vi "XW_Linearise_+_temp_comp.vi"(5 "Calib const":dbl[](array[numeric]) format="%.4f", 6 "XW2 voltage":dbl[](array[numeric]) format="%.4f", 7 "XW1 voltage":dbl[](array[numeric]) format="%.4f") -> (0 "U1":dbl[](array[numeric]) format="%.2f", 1 "V":dbl[](array[numeric]) format="%.2f", 2 "U2":dbl[](array[numeric]) format="%.2f", 3 "U":dbl[](array[numeric]) format="%.2f")   [LabVIEW 2011]
uses:
  XW calib map/XW_Map_Global.vi
  Globals/Meas_global.vi
  Globals/Dynamic_call_global.ph.vi
  <vilib>/Analysis/NI_AALBase.lvlib
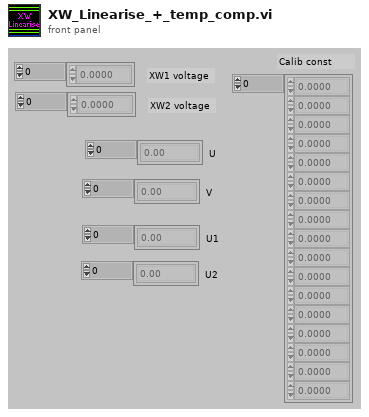
[diagram p1: front panel]
types:
  T1 = cluster{"Calib const[0]":dbl, "Calib const[1]":dbl, "Calib const[2]":dbl, "Calib const[3]":dbl, "Calib const[4]":dbl, "Calib const[5]":dbl, "Calib const[6]":dbl, "Calib const[7]":dbl, "Calib const[8]":dbl, "Calib const[9]":dbl, "Calib const[10]":dbl, "Calib const[11]":dbl, "Calib const[12]":dbl, "Calib const[13]":dbl, "Calib const[14]":dbl, "Calib const[15]":dbl, "Calib const[16]":dbl, "Calib const[17]":dbl}
  T2 = typedef "Map method.ctl" = enum16{"Triangle mesh", "Polynomial surface", "Const. Psi_eff (std.)", "Psi_eff = f(Umagn.)", "Psi_eff, k = f(Umagn.)"}
  T3 = typedef "Trimmed down TreeNode2D.ctl" = cluster{"Xmax":dbl, "Xmin":dbl, "Ymax":dbl, "Ymin":dbl, "Xc":dbl, "Yc":dbl, "ObjIndexList":i32[], "NodeQ1Index":i32, "NodeQ2Index":i32, "NodeQ3Index":i32, "NodeQ4Index":i32}
  T4 = typedef "Triangle2D.ctl" = cluster{"V10":dbl[], "V20":dbl[], "1/det":dbl, "V0":cluster{"PosVector":dbl[], "ValueVector":dbl[]}, "V1":cluster{"PosVector":dbl[], "ValueVector":dbl[]}, "V2":cluster{"PosVector":dbl[], "ValueVector":dbl[]}, "V21":dbl[]}
  T5 = enum16{"2nd component as calculated", "2nd component multipled by -1"}
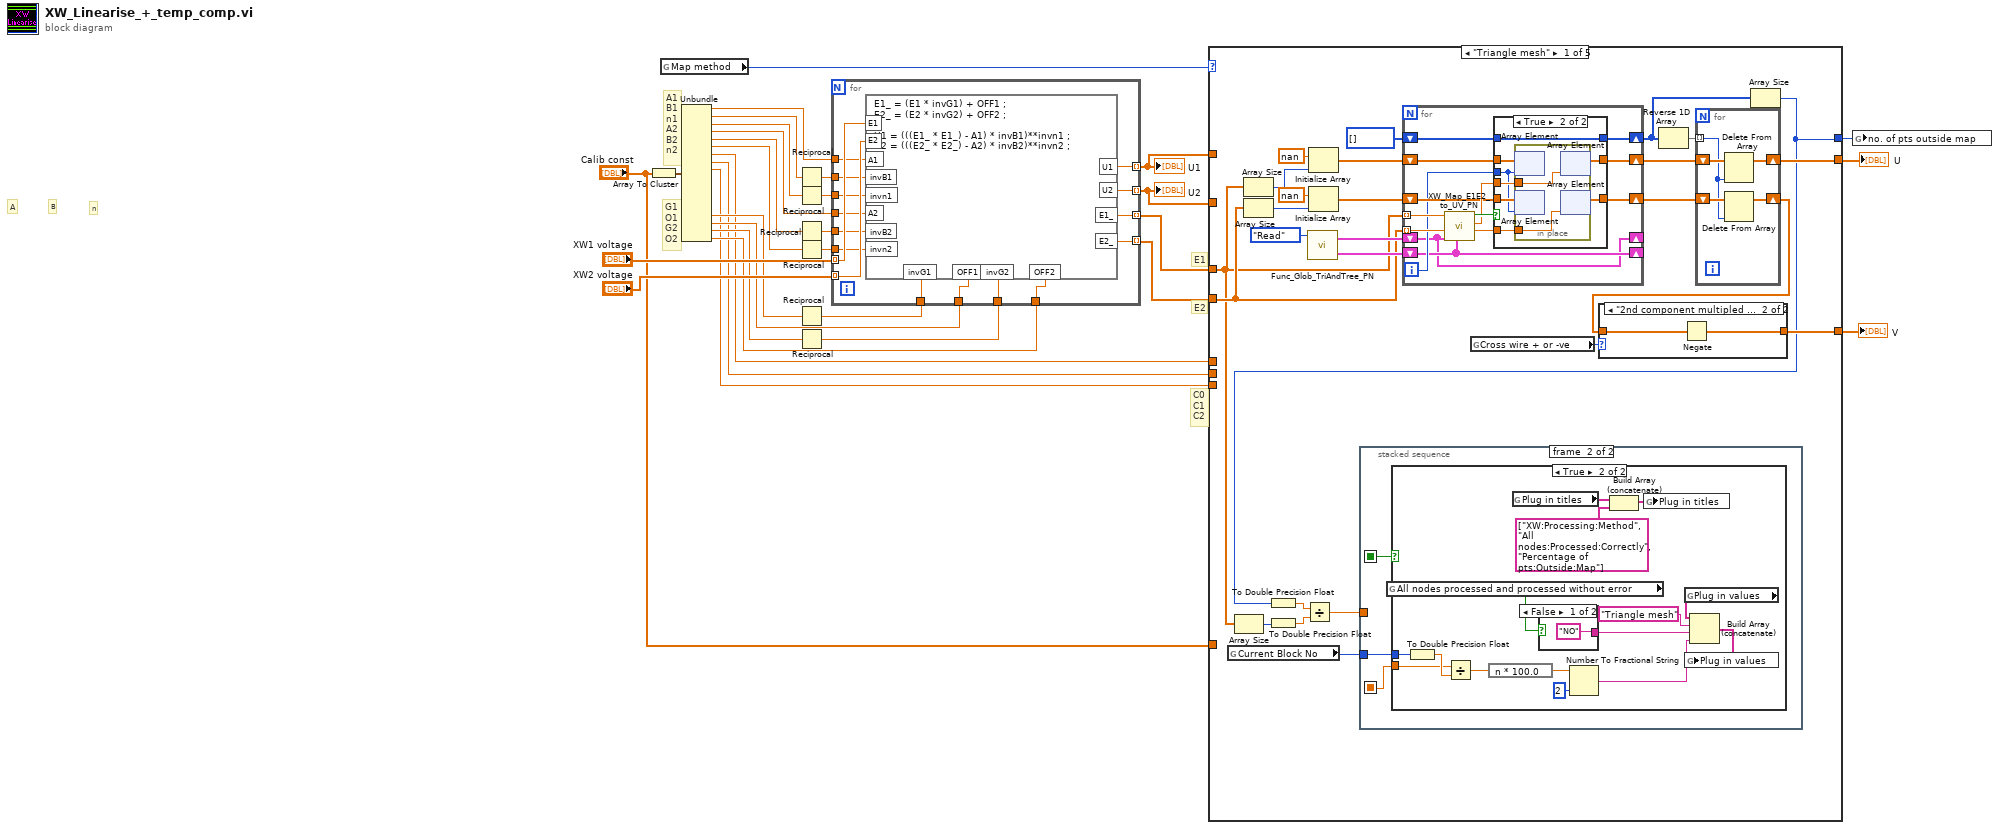
[diagram p0: block diagram]
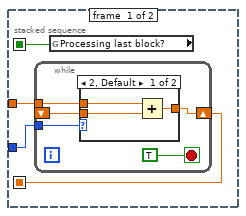
[diagram p2: hidden frame]
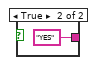
[diagram p5: hidden frame]
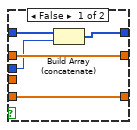
[diagram p6: hidden frame]
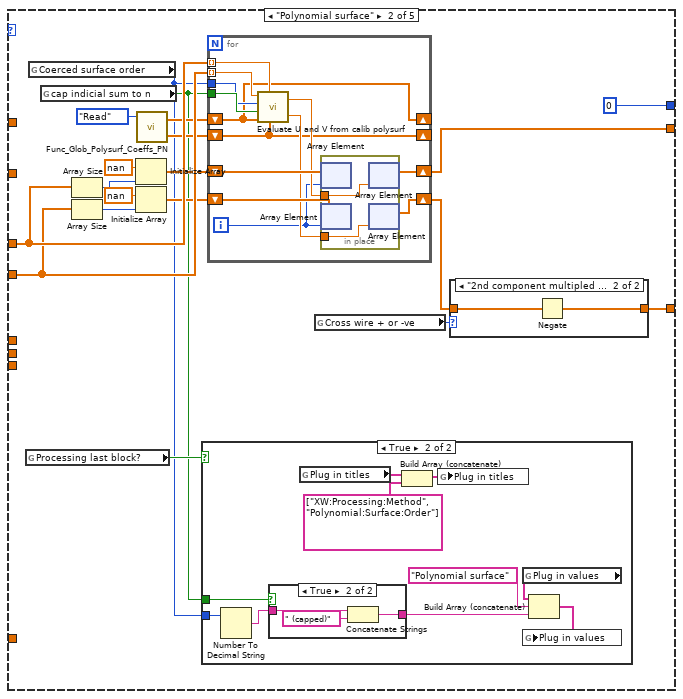
[diagram p8: hidden frame]
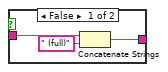
[diagram p10: hidden frame]
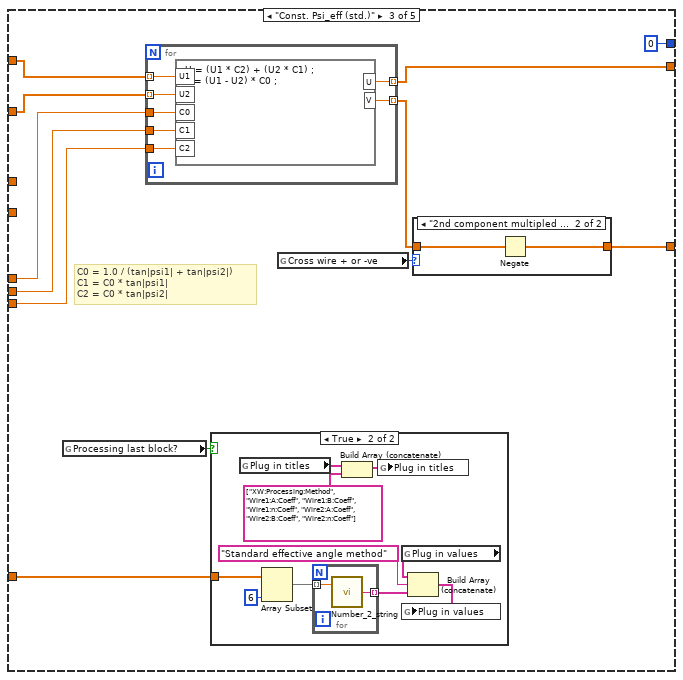
[diagram p12: hidden frame]
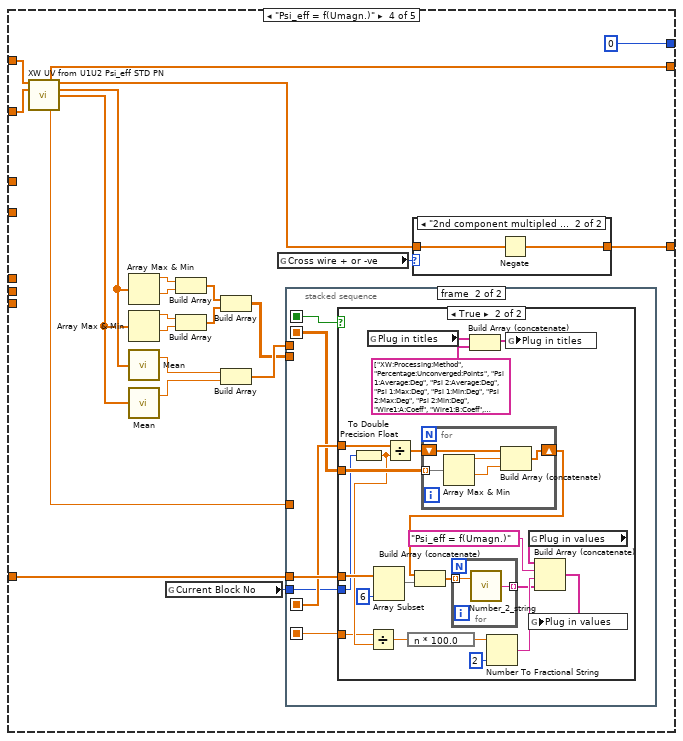
[diagram p15: hidden frame]
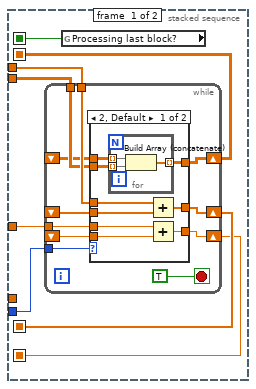
[diagram p16: hidden frame]
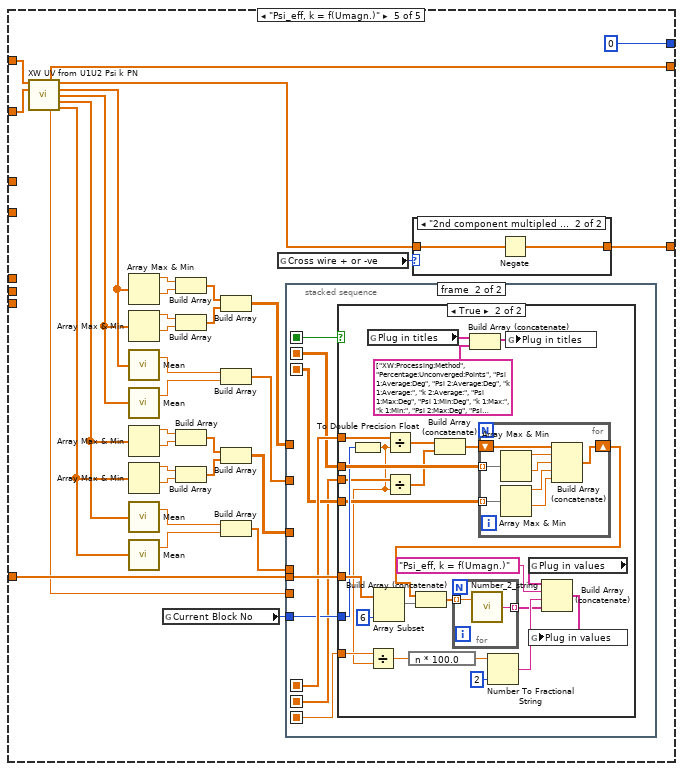
[diagram p20: hidden frame]
diagram:
  # "C0\nC1\nC2"
  # "E2"
  # "E1"
  # "G1\nO1\nG2\nO2"
  # "A1\nB1\nn1\nA2\nB2\nn2"
  # "n"
  # "B"
  # "A"
  n1 = Array To Cluster(array="Calib const") -> (cluster=w31:T1)
  n2 = global read "XW_Map_Global.vi" "Map method"() -> (w28:T2)
  n3 = Unbundle(w31) -> ("Calib const[0]"=w22:dbl, "Calib const[1]"=w16:dbl, "Calib const[2]"=w12:dbl, "Calib const[3]"=w21:dbl, "Calib const[4]"=w14:dbl, "Calib const[5]"=w10:dbl, "Calib const[6]"=w3:dbl, "Calib const[7]"=w2:dbl, "Calib const[8]"=w1:dbl, "Calib const[14]"=w8:dbl, "Calib const[15]"=w19:dbl, "Calib const[16]"=w6:dbl, "Calib const[17]"=w20:dbl)  [unwired: 5 out]
  n4 = Reciprocal(x=w16) -> (1/x=w15:dbl)
  n5 = Reciprocal(x=w12) -> (1/x=w11:dbl)
  n6 = Reciprocal(x=w14) -> (1/x=w13:dbl)
  n7 = Reciprocal(x=w10) -> (1/x=w9:dbl)
  n8 = Reciprocal(x=w8) -> (1/x=w7:dbl)
  n9 = Reciprocal(x=w6) -> (1/x=w5:dbl)
  n10 = for {
    tunnel: [w47] -> w26 mode=indexing
    tunnel: [w46] -> w25 mode=indexing
    tunnel: [w45] -> w18 mode=indexing
    tunnel: [w44] -> w17 mode=indexing
    tunnel: "XW1 voltage" -> [w43] mode=indexing
    tunnel: "XW2 voltage" -> [w42] mode=indexing
    tunnel: w22 -> [w41]
    tunnel: w15 -> [w40]
    tunnel: w11 -> [w39]
    tunnel: w21 -> [w38]
    tunnel: w13 -> [w37]
    tunnel: w9 -> [w36]
    tunnel: w20 -> [w35]
    tunnel: w5 -> [w34]
    tunnel: w19 -> [w33]
    tunnel: w7 -> [w32]
    n11 = formula code="E1_ = (E1 * invG1) + OFF1 ;\nE2_ = (E2 * invG2) + OFF2 ;\n\nU1 = (((E1_ * E1_) - A1) * invB1)**invn1 ;\nU2 = (((E2_ * E2_) - A2) * invB2)**invn2 ;"("E1"=w43, "E2"=w42, "A1"=w41, "invB1"=w40, "invn1"=w39, "A2"=w38, "invB2"=w37, "invn2"=w36, "invG1"=w32, "OFF1"=w33, "invG2"=w34, "OFF2"=w35) -> ("E1_"=w47:dbl, "E2_"=w46:dbl, "U1"=w45:dbl, "U2"=w44:dbl)
  }
  "U2" <- w17
  "U1" <- w18
  n12 = case shown="\"Triangle mesh\"" w28 {
    tunnel: w25 -> [w54 w155 _ _ _]
    tunnel: w26 -> [w50 w156 _ _ _]
    tunnel: [w60 w152 w204 w250 w355] -> w30
    tunnel: [w73 w162 w206 w236 w352] -> w29
    tunnel: [w55 0 0 0 0] -> w27
    tunnel: w18 -> [_ _ w203 w252 w357]
    tunnel: w17 -> [_ _ w202 w251 w356]
    tunnel: "Calib const" -> [_ _ w198 w232 w338]
    tunnel: w3 -> [_ _ w201 _ _]
    tunnel: w2 -> [_ _ w200 _ _]
    tunnel: w1 -> [_ _ w199 _ _]
    frame "Triangle mesh" {
      n13 = global read "Meas_global.vi" "Current Block No"() -> (w49:i32)
      n14 = Array Size(array=w50) -> (size(s)=w53:i32)
      n15 = Array Size(array=w50) -> (size(s)=w69:i32)
      n16 = Array Size(array=w54) -> (size(s)=w68:i32)
      n17 = To Double Precision Float(number=w53) -> (double precision float=w51:dbl)
      n18 = call "Func_Glob_TriAndTree_PN.vi"("Action"=enum16{"Read", "Write"}."Read") -> ("Trimmed down TreeNode array OUT"=w56:T3[], "Corrected triangles OUT"=w57:T4[])  [unwired: 2 in]
      n19 = Initialize Array(nan ("element"), w69) -> (w66:dbl[])
      n20 = Initialize Array(nan ("element"), w68) -> (w67:dbl[])
      n21 = for {
        tunnel: w50 -> [w125] mode=indexing
        tunnel: w54 -> [w124] mode=indexing
        shift-right: [w113] -> w59
        shift-left: i32[] [] -> [w112]
        shift-right: [w120] -> w64
        shift-left: w66 -> [w119]
        shift-right: [w117] -> w63
        shift-left: w67 -> [w118]
        shift-right: [w114] -> _
        shift-left: w57 -> [w114]
        shift-right: [w115] -> _
        shift-left: w56 -> [w115]
        i -> [w116]
        n22 = call "XW_Map_E1E2_to_UV_PN.vi"("Trimmed down TreeNode array"=w115, "Triangulated XW Calib Map Mesh"=w114, "(E2 / G2) + O2 (Volts)"=w124, "(E1 / G1) + O1 (Volts)"=w125) -> ("V (m/s)"=w121:dbl, "U (m/s)"=w122:dbl, "Voltages are inside calibrated region"=w123:bool)  [unwired: 5 out]
        n23 = case shown="True" w123 {
          tunnel: w122 -> [_ w134]
          tunnel: w112 -> [w126 w138]
          tunnel: [w127 w138] -> w113
          tunnel: w121 -> [_ w133]
          tunnel: [w130 w136] -> w120
          tunnel: w119 -> [w130 w137]
          tunnel: w118 -> [w129 w135]
          tunnel: [w129 w132] -> w117
          tunnel: w116 -> [w128 w131]
          frame False {
            n24 = Build Array (concatenate)(w126, w128) -> (w127:i32[])
          }
          frame True {
            n25 = in-place {
              in-place-border: w134 -> [w140]
              in-place-border: w133 -> [w139]
              n26 = in-place-array #1(w137, w131) -> ()  [unwired: 1 out]
              n27 = in-place-array #2(w135, w131) -> ()  [unwired: 1 out]
              n28 = in-place-array #1(w140) -> (w136:dbl[])  [unwired: 1 out]
              n29 = in-place-array #2(w139) -> (w132:dbl[])  [unwired: 1 out]
            }
          }
        }
      }
      n30 = global read "Meas_global.vi" "Cross wire + or -ve"() -> (w72:T5)
      n31 = Reverse 1D Array(array=w59) -> (reversed array=w62:i32[])
      n32 = for {
        shift-right: [w108] -> w60
        shift-left: w64 -> [w111]
        shift-right: [w109] -> w61
        shift-left: w63 -> [w110]
        tunnel: w62 -> [w107] mode=indexing
        n33 = Delete From Array(array=w111, index=w107) -> (array with subset deleted=w108:dbl[])  [unwired: 1 in, 1 out]
        n34 = Delete From Array(array=w110, index=w107) -> (array with subset deleted=w109:dbl[])  [unwired: 1 in, 1 out]
      }
      n35 = case shown="\"2nd component multipled by -1\"" w72 {
        tunnel: [w141 w143] -> w73
        tunnel: w61 -> [w141 w142]
        frame "2nd component as calculated" {
        }
        frame "2nd component multipled by -1" {
          n36 = Negate(x=w142) -> (-x=w143:dbl[])
        }
      }
      n37 = Array Size(array=w59) -> (size(s)=w55:i32)
      n38 = To Double Precision Float(number=w55) -> (double precision float=w52:dbl)
      n39 = Divide(x=w52, y=w51) -> (x/y=w48:dbl)
      n40 = stacked-sequence {
        seq-local: [w77 _] -> [_ w87]
        seq-local: [w76 _] -> [_ w89]
        tunnel: w49 -> [w75 w88]
        tunnel: w48 -> [w74 _]
        frame #0 {
          n41 = while {
            shift-right: [w82] -> w77
            shift-left: _ -> [w79]
            tunnel: w75 -> [w80]
            tunnel: w74 -> [w78]
            stop <- TRUE stop-if-true
            n42 = case shown="2, Default" w80 {
              tunnel: w79 -> [w84 _]
              tunnel: [w85 w86] -> w82
              tunnel: w78 -> [w83 w86]
              frame 2, Default {
                n43 = Add(x=w83, y=w84) -> (x+y=w85:dbl)
              }
              frame 1 {
              }
            }
          }
          n44 = global read "Meas_global.vi" "Processing last block?"() -> (w76:bool)
        }
        frame #1 {
          n45 = case shown="True" w89 {
            tunnel: w88 -> [_ w104]
            tunnel: w87 -> [_ w101]
            frame False {
            }
            frame True {
              n46 = global read "XW_Map_Global.vi" "All nodes processed and processed without error"() -> (w99:bool)
              n47 = To Double Precision Float(number=w104) -> (double precision float=w102:dbl)
              n48 = Divide(x=w101, y=w102) -> (x/y=w91:dbl)
              n49 = expression code="n * 100.0"(w91) -> (w90:dbl)
              n50 = global read "Dynamic_call_global.ph.vi" "Plug in titles"() -> (w95:string[])
              n51 = case shown="False" w99 {
                tunnel: ["NO" "YES"] -> w100
                frame False {
                }
                frame True {
                }
              }
              n52 = Number To Fractional String(number=w90, precision (6)=i16 2) -> (F-format string=w92:string)  [unwired: 2 out]
              n53 = Build Array (concatenate)(w95, string[] ["XW:Processing:Method", "All nodes:Processed:Correctly", "Percentage of pts:Outside:Map"] ("array")) -> (w93:string[])
              n54 = global write "Dynamic_call_global.ph.vi" "Plug in titles"(w93) -> ()
              n55 = global read "Dynamic_call_global.ph.vi" "Plug in values"() -> (w97:string[])
              n56 = Build Array (concatenate)(w97, "Triangle mesh", w100, w92) -> (w94:string[])
              n57 = global write "Dynamic_call_global.ph.vi" "Plug in values"(w94) -> ()
            }
          }
        }
      }
    }
    frame "Polynomial surface" {
      n58 = global read "Meas_global.vi" "Processing last block?"() -> (w146:bool)
      n59 = global read "XW_Map_Global.vi" "Coerced surface order"() -> (w145:i32)
      n60 = global read "XW_Map_Global.vi" "cap indicial sum to n"() -> (w144:bool)
      n61 = Array Size(array=w156) -> (size(s)=w158:i32)
      n62 = Array Size(array=w155) -> (size(s)=w157:i32)
      n63 = Initialize Array(nan ("element"), w158) -> (w154:dbl[])
      n64 = Initialize Array(nan ("element"), w157) -> (w153:dbl[])
      n65 = call "Func_Glob_Polysurf_Coeffs_PN.vi"("Action"=enum16{"Read", "Write"}."Read") -> ("alpha(rad) coeffs OUT"=w148:dbl[], "Ucal coeffs OUT"=w149:dbl[])  [unwired: 2 in]
      n66 = case shown="True" w146 {
        tunnel: w145 -> [_ w165]
        tunnel: w144 -> [_ w163]
        frame False {
        }
        frame True {
          n67 = Number To Decimal String(number=w165) -> (decimal integer string=w164:string)  [unwired: 1 out]
          n68 = case shown="True" w163 {
            tunnel: [w173 w176] -> w166
            tunnel: w164 -> [w175 w178]
            frame False {
              n69 = Concatenate Strings(w175, " (full)") -> (w173:string)
            }
            frame True {
              n70 = Concatenate Strings(w178, " (capped)") -> (w176:string)
            }
          }
          n71 = global read "Dynamic_call_global.ph.vi" "Plug in titles"() -> (w170:string[])
          n72 = Build Array (concatenate)(w170, string[] ["XW:Processing:Method", "Polynomial:Surface:Order"] ("array")) -> (w172:string[])
          n73 = global write "Dynamic_call_global.ph.vi" "Plug in titles"(w172) -> ()
          n74 = global read "Dynamic_call_global.ph.vi" "Plug in values"() -> (w168:string[])
          n75 = Build Array (concatenate)(w168, "Polynomial surface", w166) -> (w171:string[])
          n76 = global write "Dynamic_call_global.ph.vi" "Plug in values"(w171) -> ()
        }
      }
      n77 = for {
        tunnel: w156 -> [w191] mode=indexing
        tunnel: w155 -> [w190] mode=indexing
        tunnel: w144 -> [w189]
        shift-right: [w187] -> w151
        shift-left: w153 -> [w185]
        shift-right: [w188] -> w152
        shift-left: w154 -> [w186]
        tunnel: w145 -> [w181]
        shift-right: [w180] -> _
        shift-left: w148 -> [w180]
        shift-right: [w179] -> _
        shift-left: w149 -> [w179]
        i -> [w182]
        n78 = call "Evaluate U and V from calib polysurf.vi"("alpha(rad) coeffs"=w180, "E1 / G1 + O1"=w191, "Ucal coeffs"=w179, "cap indicial sum to n"=w189, "surface order (n)"=w181, "E2 / G2 + O2"=w190) -> ("V (m/s)"=w184:dbl, "U (m/s)"=w183:dbl)
        n79 = in-place {
          in-place-border: w183 -> [w193]
          in-place-border: w184 -> [w192]
          n80 = in-place-array #3(w186, w182) -> ()  [unwired: 1 out]
          n81 = in-place-array #4(w185, w182) -> ()  [unwired: 1 out]
          n82 = in-place-array #3(w193) -> (w188:dbl[])  [unwired: 1 out]
          n83 = in-place-array #4(w192) -> (w187:dbl[])  [unwired: 1 out]
        }
      }
      n84 = global read "Meas_global.vi" "Cross wire + or -ve"() -> (w161:T5)
      n85 = case shown="\"2nd component multipled by -1\"" w161 {
        tunnel: [w194 w196] -> w162
        tunnel: w151 -> [w194 w195]
        frame "2nd component as calculated" {
        }
        frame "2nd component multipled by -1" {
          n86 = Negate(x=w195) -> (-x=w196:dbl[])
        }
      }
    }
    frame "Const. Psi_eff (std.)" {
      # "C0 = 1.0 / (tan|psi1| + tan|psi2|)\nC1 = C0 * tan|psi1|\nC2 = C0 * tan|psi2|"
      n87 = global read "Meas_global.vi" "Processing last block?"() -> (w197:bool)
      n88 = for {
        tunnel: [w227] -> w205 mode=indexing
        tunnel: [w226] -> w204 mode=indexing
        tunnel: w203 -> [w225] mode=indexing
        tunnel: w202 -> [w224] mode=indexing
        tunnel: w201 -> [w223]
        tunnel: w200 -> [w222]
        tunnel: w199 -> [w221]
        n89 = formula code="U = (U1 * C2) + (U2 * C1) ;\nV = (U1 - U2) * C0 ;"("U1"=w225, "U2"=w224, "C1"=w222, "C2"=w221, "C0"=w223) -> ("U"=w226:dbl, "V"=w227:dbl)
      }
      n90 = case shown="True" w197 {
        tunnel: w198 -> [_ w212]
        frame False {
        }
        frame True {
          n91 = global read "Dynamic_call_global.ph.vi" "Plug in titles"() -> (w216:string[])
          n92 = Array Subset(array=w212, length=6) -> (w211:dbl[])  [unwired: 1 in]
          n93 = for {
            tunnel: w211 -> [w220] mode=indexing
            tunnel: [w219] -> w215 mode=indexing
            n94 = call "Number_2_string.vi"("number"=w220) -> ("String"=w219:string)  [unwired: 1 in]
          }
          n95 = Build Array (concatenate)(w216, string[] ["XW:Processing:Method", "Wire1:A:Coeff", "Wire1:B:Coeff", "Wire1:n:Coeff", "Wire2:A:Coeff", "Wire2:B:Coeff", "Wire2:n:Coeff"] ("array")) -> (w218:string[])
          n96 = global write "Dynamic_call_global.ph.vi" "Plug in titles"(w218) -> ()
          n97 = global read "Dynamic_call_global.ph.vi" "Plug in values"() -> (w210:string[])
          n98 = Build Array (concatenate)(w210, "Standard effective angle method", w215) -> (w217:string[])
          n99 = global write "Dynamic_call_global.ph.vi" "Plug in values"(w217) -> ()
        }
      }
      n100 = global read "Meas_global.vi" "Cross wire + or -ve"() -> (w207:T5)
      n101 = case shown="\"2nd component multipled by -1\"" w207 {
        tunnel: [w228 w230] -> w206
        tunnel: w205 -> [w228 w229]
        frame "2nd component as calculated" {
        }
        frame "2nd component multipled by -1" {
          n102 = Negate(x=w229) -> (-x=w230:dbl[])
        }
      }
    }
    frame "Psi_eff = f(Umagn.)" {
      n103 = call "XW UV from U1U2 Psi_eff STD PN.vi"("U1cal (m/s)"=w252, "U2cal (m/s)"=w251) -> ("U (m/s)"=w250:dbl[], "V (m/s)"=w237:dbl[], "Psi1 (deg)"=w248:dbl[], "Psi2 (deg)"=w247:dbl[], "Unconverged points (fraction)"=w231:dbl)  [unwired: 9 out]
      n104 = Array Max & Min(array=w248) -> (max value=w243:dbl, min value=w244:dbl)  [unwired: 2 out]
      n105 = Array Max & Min(array=w247) -> (max value=w242:dbl, min value=w241:dbl)  [unwired: 2 out]
      n106 = call <vilib>:"Mean.vi"("X"=w248) -> ("mean"=w246:dbl)  [unwired: 1 out]
      n107 = call <vilib>:"Mean.vi"("X"=w247) -> ("mean"=w245:dbl)  [unwired: 1 out]
      n108 = global read "Meas_global.vi" "Current Block No"() -> (w235:i32)
      n109 = Build Array(w243, w244) -> (w239:dbl[])
      n110 = Build Array(w242, w241) -> (w240:dbl[])
      n111 = Build Array(w239, w240) -> (w233:dbl[][])
      n112 = Build Array(w246, w245) -> (w234:dbl[])
      n113 = global read "Meas_global.vi" "Cross wire + or -ve"() -> (w238:T5)
      n114 = stacked-sequence {
        seq-local: [w258 _] -> [_ w291]
        seq-local: [w256 _] -> [_ w289]
        seq-local: [w257 _] -> [_ w290]
        seq-local: [w253 _] -> [_ w287]
        tunnel: w234 -> [w260 _]
        tunnel: w233 -> [w259 _]
        tunnel: w232 -> [_ w292]
        tunnel: w235 -> [w255 w288]
        tunnel: w231 -> [w254 _]
        frame #0 {
          n115 = while {
            shift-right: [w269] -> w258
            shift-left: _ -> [w270]
            tunnel: w260 -> [w271]
            shift-right: [w267] -> w256
            shift-left: _ -> [w265]
            tunnel: w259 -> [w266]
            tunnel: w255 -> [w264]
            shift-right: [w261] -> w253
            shift-left: _ -> [w263]
            tunnel: w254 -> [w262]
            stop <- TRUE stop-if-true
            n116 = case shown="2, Default" w264 {
              tunnel: w271 -> [w280 w286]
              tunnel: w270 -> [w279 _]
              tunnel: [w278 w286] -> w269
              tunnel: [w275 w285] -> w267
              tunnel: w266 -> [w276 w285]
              tunnel: w265 -> [w277 _]
              tunnel: [w274 w284] -> w261
              tunnel: w263 -> [w273 _]
              tunnel: w262 -> [w272 w284]
              frame 2, Default {
                n117 = for {
                  tunnel: w277 -> [w283] mode=indexing
                  tunnel: w276 -> [w282] mode=indexing
                  tunnel: [w281] -> w275 mode=indexing
                  n118 = Build Array (concatenate)(w283, w282) -> (w281:dbl[])
                }
                n119 = Add(x=w280, y=w279) -> (x+y=w278:dbl[])
                n120 = Add(x=w272, y=w273) -> (x+y=w274:dbl)
              }
              frame 1 {
              }
            }
          }
          n121 = global read "Meas_global.vi" "Processing last block?"() -> (w257:bool)
        }
        frame #1 {
          n122 = case shown="True" w290 {
            tunnel: w291 -> [_ w311]
            tunnel: w292 -> [_ w308]
            tunnel: w288 -> [_ w302]
            tunnel: w289 -> [_ w305]
            tunnel: w287 -> [_ w295]
            frame False {
            }
            frame True {
              n123 = To Double Precision Float(number=w302) -> (double precision float=w296:dbl)
              n124 = global read "Dynamic_call_global.ph.vi" "Plug in titles"() -> (w312:string[])
              n125 = Divide(x=w295, y=w296) -> (x/y=w294:dbl)
              n126 = Array Subset(array=w308, length=6) -> (w307:dbl[])  [unwired: 1 in]
              n127 = Divide(x=w311, y=w296) -> (x/y=w304:dbl[])
              n128 = expression code="n * 100.0"(w294) -> (w293:dbl)
              n129 = for {
                tunnel: w305 -> [w319] mode=indexing
                shift-right: [w315] -> w303
                shift-left: w304 -> [w318]
                n130 = Array Max & Min(array=w319) -> (max value=w317:dbl, min value=w316:dbl)  [unwired: 2 out]
                n131 = Build Array (concatenate)(w318, w317, w316) -> (w315:dbl[])
              }
              n132 = Build Array (concatenate)(w303, w307) -> (w306:dbl[])
              n133 = for {
                tunnel: w306 -> [w321] mode=indexing
                tunnel: [w320] -> w297 mode=indexing
                n134 = call "Number_2_string.vi"("number"=w321) -> ("String"=w320:string)  [unwired: 1 in]
              }
              n135 = Build Array (concatenate)(w312, string[] ["XW:Processing:Method", "Percentage:Unconverged:Points", "Psi 1:Average:Deg", "Psi 2:Average:Deg", "Psi 1:Max:Deg", "Psi 1:Min:Deg", "Psi 2:Max:Deg", "Psi 2:Min:Deg", "Wire1:A:Coeff", "Wire1:B:Coeff", "Wire1:n:Coeff", "Wire2:A:Coeff", "Wire2:B:Coeff", "Wire2:n:Coeff"] ("array")) -> (w314:string[])
              n136 = Number To Fractional String(number=w293, precision (6)=i16 2) -> (F-format string=w298:string)  [unwired: 2 out]
              n137 = global write "Dynamic_call_global.ph.vi" "Plug in titles"(w314) -> ()
              n138 = global read "Dynamic_call_global.ph.vi" "Plug in values"() -> (w301:string[])
              n139 = Build Array (concatenate)(w301, "Psi_eff = f(Umagn.)", w298, w297) -> (w313:string[])
              n140 = global write "Dynamic_call_global.ph.vi" "Plug in values"(w313) -> ()
            }
          }
        }
      }
      n141 = case shown="\"2nd component multipled by -1\"" w238 {
        tunnel: [w322 w324] -> w236
        tunnel: w237 -> [w322 w323]
        frame "2nd component as calculated" {
        }
        frame "2nd component multipled by -1" {
          n142 = Negate(x=w323) -> (-x=w324:dbl[])
        }
      }
    }
    frame "Psi_eff, k = f(Umagn.)" {
      n143 = call "XW UV from U1U2 Psi k PN.vi"("U1cal (m/s)"=w357, "U2cal (m/s)"=w356) -> ("U (m/s)"=w355:dbl[], "V (m/s)"=w353:dbl[], "Psi1 (deg)"=w343:dbl[], "Psi2 (deg)"=w342:dbl[], "k1"=w329:dbl[], "Unconverged points (fraction)"=w325:dbl, "k2"=w328:dbl[])  [unwired: 7 out]
      n144 = Array Max & Min(array=w343) -> (max value=w348:dbl, min value=w349:dbl)  [unwired: 2 out]
      n145 = Array Max & Min(array=w342) -> (max value=w347:dbl, min value=w346:dbl)  [unwired: 2 out]
      n146 = call <vilib>:"Mean.vi"("X"=w343) -> ("mean"=w351:dbl)  [unwired: 1 out]
      n147 = call <vilib>:"Mean.vi"("X"=w342) -> ("mean"=w350:dbl)  [unwired: 1 out]
      n148 = Array Max & Min(array=w329) -> (max value=w333:dbl, min value=w332:dbl)  [unwired: 2 out]
      n149 = Array Max & Min(array=w328) -> (max value=w334:dbl, min value=w335:dbl)  [unwired: 2 out]
      n150 = call <vilib>:"Mean.vi"("X"=w329) -> ("mean"=w330:dbl)  [unwired: 1 out]
      n151 = call <vilib>:"Mean.vi"("X"=w328) -> ("mean"=w331:dbl)  [unwired: 1 out]
      n152 = global read "Meas_global.vi" "Current Block No"() -> (w339:i32)
      n153 = Build Array(w348, w349) -> (w344:dbl[])
      n154 = Build Array(w347, w346) -> (w345:dbl[])
      n155 = Build Array(w333, w332) -> (w337:dbl[])
      n156 = Build Array(w334, w335) -> (w336:dbl[])
      n157 = Build Array(w344, w345) -> (w341:dbl[][])
      n158 = Build Array(w351, w350) -> (w340:dbl[])
      n159 = Build Array(w337, w336) -> (w326:dbl[][])
      n160 = Build Array(w330, w331) -> (w327:dbl[])
      n161 = global read "Meas_global.vi" "Cross wire + or -ve"() -> (w354:T5)
      n162 = stacked-sequence {
        seq-local: [w368 _] -> [_ w420]
        seq-local: [w366 _] -> [_ w418]
        seq-local: [w367 _] -> [_ w419]
        seq-local: [w362 _] -> [_ w416]
        seq-local: [w361 _] -> [_ w415]
        seq-local: [w359 _] -> [_ w414]
        tunnel: w340 -> [w370 _]
        tunnel: w341 -> [w369 _]
        tunnel: w338 -> [_ w421]
        tunnel: w339 -> [w365 w417]
        tunnel: w327 -> [w364 _]
        tunnel: w326 -> [w363 _]
        tunnel: w325 -> [w360 _]
        frame #0 {
          n163 = while {
            shift-right: [w385] -> w368
            shift-left: _ -> [w386]
            tunnel: w370 -> [w387]
            shift-right: [w383] -> w366
            shift-left: _ -> [w381]
            tunnel: w369 -> [w382]
            tunnel: w365 -> [w380]
            tunnel: w364 -> [w379]
            shift-right: [w377] -> w361
            shift-left: _ -> [w378]
            shift-right: [w376] -> w362
            shift-left: _ -> [w375]
            tunnel: w363 -> [w374]
            tunnel: w360 -> [w373]
            shift-right: [w371] -> w359
            shift-left: _ -> [w372]
            stop <- TRUE stop-if-true
            n164 = case shown="2, Default" w380 {
              tunnel: w387 -> [w402 w413]
              tunnel: w386 -> [w397 _]
              tunnel: [w401 w413] -> w385
              tunnel: [w398 w412] -> w383
              tunnel: w382 -> [w399 w412]
              tunnel: w381 -> [w400 _]
              tunnel: w379 -> [w396 w410]
              tunnel: w378 -> [w395 _]
              tunnel: [w394 w410] -> w377
              tunnel: [w393 w411] -> w376
              tunnel: w375 -> [w392 _]
              tunnel: w374 -> [w391 w411]
              tunnel: w373 -> [w390 w409]
              tunnel: [w389 w409] -> w371
              tunnel: w372 -> [w388 _]
              frame 2, Default {
                n165 = for {
                  tunnel: w400 -> [w408] mode=indexing
                  tunnel: w399 -> [w407] mode=indexing
                  tunnel: [w406] -> w398 mode=indexing
                  n166 = Build Array (concatenate)(w408, w407) -> (w406:dbl[])
                }
                n167 = for {
                  tunnel: w392 -> [w403] mode=indexing
                  tunnel: w391 -> [w405] mode=indexing
                  tunnel: [w404] -> w393 mode=indexing
                  n168 = Build Array (concatenate)(w403, w405) -> (w404:dbl[])
                }
                n169 = Add(x=w402, y=w397) -> (x+y=w401:dbl[])
                n170 = Add(x=w396, y=w395) -> (x+y=w394:dbl[])
                n171 = Add(x=w390, y=w388) -> (x+y=w389:dbl)
              }
              frame 1 {
              }
            }
          }
          n172 = global read "Meas_global.vi" "Processing last block?"() -> (w367:bool)
        }
        frame #1 {
          n173 = case shown="True" w419 {
            tunnel: w420 -> [_ w444]
            tunnel: w421 -> [_ w442]
            tunnel: w417 -> [_ w438]
            tunnel: w418 -> [_ w439]
            tunnel: w416 -> [_ w437]
            tunnel: w415 -> [_ w436]
            tunnel: w414 -> [_ w425]
            frame False {
            }
            frame True {
              n174 = To Double Precision Float(number=w438) -> (double precision float=w424:dbl)
              n175 = global read "Dynamic_call_global.ph.vi" "Plug in titles"() -> (w445:string[])
              n176 = Divide(x=w425, y=w424) -> (x/y=w423:dbl)
              n177 = Array Subset(array=w442, length=6) -> (w441:dbl[])  [unwired: 1 in]
              n178 = Divide(x=w444, y=w424) -> (x/y=w435:dbl[])
              n179 = Divide(x=w436, y=w424) -> (x/y=w434:dbl[])
              n180 = expression code="n * 100.0"(w423) -> (w422:dbl)
              n181 = Build Array (concatenate)(w435, w434) -> (w433:dbl[])
              n182 = Build Array (concatenate)(w445, string[] ["XW:Processing:Method", "Percentage:Unconverged:Points", "Psi 1:Average:Deg", "Psi 2:Average:Deg", "k 1:Average:", "k 2:Average:", "Psi 1:Max:Deg", "Psi 1:Min:Deg", "k 1:Max:", "k 1:Min:", "Psi 2:Max:Deg", "Psi 2:Min:Deg", "k 2:Max:", "k 2:Min:", "Wire1:A:Coeff", "Wire1:B:Coeff", "Wire1:n:Coeff", "Wire2:A:Coeff", "Wire2:B:Coeff", "Wire2:n:Coeff"] ("array")) -> (w447:string[])
              n183 = for {
                tunnel: w439 -> [w455] mode=indexing
                shift-right: [w451] -> w429
                shift-left: w433 -> [w454]
                tunnel: w437 -> [w448] mode=indexing
                n184 = Array Max & Min(array=w455) -> (max value=w453:dbl, min value=w452:dbl)  [unwired: 2 out]
                n185 = Array Max & Min(array=w448) -> (max value=w449:dbl, min value=w450:dbl)  [unwired: 2 out]
                n186 = Build Array (concatenate)(w454, w453, w452, w449, w450) -> (w451:dbl[])
              }
              n187 = Build Array (concatenate)(w429, w441) -> (w440:dbl[])
              n188 = for {
                tunnel: w440 -> [w457] mode=indexing
                tunnel: [w456] -> w427 mode=indexing
                n189 = call "Number_2_string.vi"("number"=w457) -> ("String"=w456:string)  [unwired: 1 in]
              }
              n190 = Number To Fractional String(number=w422, precision (6)=i16 2) -> (F-format string=w428:string)  [unwired: 2 out]
              n191 = global write "Dynamic_call_global.ph.vi" "Plug in titles"(w447) -> ()
              n192 = global read "Dynamic_call_global.ph.vi" "Plug in values"() -> (w431:string[])
              n193 = Build Array (concatenate)(w431, "Psi_eff, k = f(Umagn.)", w428, w427) -> (w446:string[])
              n194 = global write "Dynamic_call_global.ph.vi" "Plug in values"(w446) -> ()
            }
          }
        }
      }
      n195 = case shown="\"2nd component multipled by -1\"" w354 {
        tunnel: [w458 w460] -> w352
        tunnel: w353 -> [w458 w459]
        frame "2nd component as calculated" {
        }
        frame "2nd component multipled by -1" {
          n196 = Negate(x=w459) -> (-x=w460:dbl[])
        }
      }
    }
  }
  "U" <- w30
  "V" <- w29
  n197 = global write "XW_Map_Global.vi" "no. of pts outside map"(w27) -> ()
